vi "Find.vi"(8 "error in (no error)":errorcluster, 11 "component objects":refnum<class>[](array[class])) -> (0 "error out":errorcluster, 2 "found?":bool, 3 "Plugin Thread":refnum<class "Plugin Thread.lvclass">)   [LabVIEW 2017, in "DSF Core.lvlib" / "Plugin Thread.lvclass"]
uses:
  Plugin Thread.lvclass
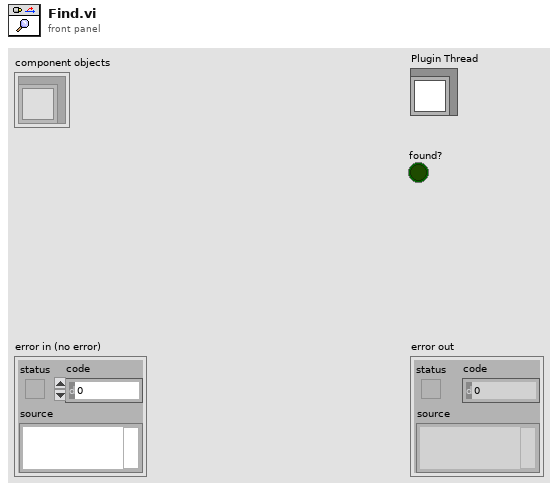
[diagram p1: front panel]
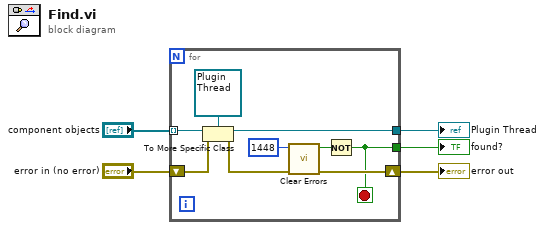
[diagram p0: block diagram]
diagram:
  n1 = for {
    tunnel: "component objects" -> [w13] mode=indexing
    shift-right: [w10] -> w2
    shift-left: "error in (no error)" -> [w9]
    tunnel: [w7] -> w1
    tunnel: [w6] -> w3
    stop <- w7 stop-if-true
    n2 = To More Specific Class(target class=refnum<class "Plugin Thread.lvclass"> refnum ("DSF.Engine.lvlib:Transceiver"), reference=w13, error in=w9) -> (specific class reference=w6:refnum<class "Plugin Thread.lvclass">, error out=w11:errorcluster)
    n3 = call <vilib>:"Clear Errors.vi"("error in (no error)"=w11, "specific error code to clear (0: all)"=1448) -> ("error out"=w10:errorcluster, "specific error cleared?"=w8:bool)  [unwired: 4 in]
    n4 = Not(x=w8) -> (.not. x?=w7:bool)
  }
  "error out" <- w2
  "Plugin Thread" <- w3
  "found?" <- w1
